vi "VisualizeTriggerTiming.vi"(1 "ExitExternalPrograms":refnum<notifier>, 2 "Pulse Settings":T1={"Pulse Length(ms)"=7.0, "DIO0Offset(ms)"=1.0, "DIO1 Pulse time (ms)"=2.0, "DIO2 Pulse time (ms) 2"=30.0, "DIO3 Pulse time (ms) 3"=0.0, "EnableDIO3"=FALSE, "EnableDIO2"=TRUE, "EnableDIO1"=TRUE}, 3 "Exposure Time (ms)":dbl=4.0, 4 "ReadoutTime":dbl=1.0, 5 "error in (no error)":errorcluster) -> (19 "error out":errorcluster)   [LabVIEW 2021]
doc: "This VI doest the same as DOconfigureCustomPattern but With a different Front panel. It is custom-made for the IAF Cytometer application"
uses:
  AD2_WFG_SDK_class/AD2TriggerSources.ctl
  AD2_SDK_class/AD2_SDK.lvclass
panel:
  in  "Tab Control":enum32{"Helper", "Ilustration"}(tab)
  out "Waveform Graph":dbl[][](graph)=[[0.0, 0.0, 0.0, 1.0, 1.0, 1.0, 1.0, 1.0, 1.0, 1.0, 0.0, 0.0, 0.0, 0.0, 0.0, 0.0, 0.0, 0.0, 0.0, 0.0, 0.0, 0.0, 0.0, 0.0, 0.0, 0.0, 0.0, 0.0, 0.0, 0.0, 0.0, 1.0, 1.0, 1.0, 1.0, 1.0, 1.0, 1.0, 0.0, 0.0, 0.0, 0.0, 0.0, 0.0], [0.0, 0.0, 1.1, 1.1, 1.1, 1.1, 1.1, 1.1, 1.1, 0.0, 0.0, 0.0, 0.0, 0.0, 0.0, 0.0, 0.0, 0.0, 0.0, 0.0, 0.0, 0.0, 0.0, 0.0, 0.0, 0.0, 0.0, 0.0, 0.0, 0.0, 0.0, 0.0, 0.0, 0.0, 0.0, 0.0, 0.0, 0.0, 0.0, 0.0, 0.0, 0.0, 0.0, 0.0], [0.0, 0.0, 0.0, 0.0, 0.0, 0.0, 0.0, 0.0, 0.0, 0.0, 0.0, 0.0, 0.0, 0.0, 0.0, 0.0, 0.0, 0.0, 0.0, 0.0, 0.0, 0.0, 0.0, 0.0, 0.0, 0.0, 0.0, 0.0, 0.0, 0.0, 1.2, 1.2, 1.2, 1.2, 1.2, 1.2, 1.2, 0.0, 0.0, 0.0, 0.0, 0.0, 0.0, 0.0], [0.0, 0.0, 0.0, 0.0, 0.0, 0.0, 0.0, 0.0, 0.0, 0.0, 0.0, 0.0, 0.0, 0.0, 0.0, 0.0, 0.0, 0.0, 0.0, 0.0, 0.0, 0.0, 0.0, 0.0, 0.0, 0.0, 0.0, 0.0, 0.0, 0.0, 0.0, 0.0, 0.0, 0.0, 0.0, 0.0, 0.0, 0.0, 0.0, 0.0, 0.0, 0.0, 0.0, 0.0], [0.0, 0.0, 0.0, 1.4, 1.4, 1.4, 1.4, 0.0, 0.0, 0.0, 0.0, 0.0, 0.0, 0.0, 0.0, 0.0, 0.0, 0.0, 0.0, 0.0, 0.0, 0.0, 0.0, 0.0, 0.0, 0.0, 0.0, 0.0, 0.0, 0.0, 0.0, 1.4, 1.4, 1.4, 1.4, 0.0, 0.0, 0.0, 0.0, 0.0, 0.0, 0.0, 0.0, 0.0], [0.0, 0.0, 0.0, 0.0, 0.0, 0.0, 0.0, 1.5, 0.0, 0.0, 0.0, 0.0, 0.0, 0.0, 0.0, 0.0, 0.0, 0.0, 0.0, 0.0, 0.0, 0.0, 0.0, 0.0, 0.0, 0.0, 0.0, 0.0, 0.0, 0.0, 0.0, 0.0, 0.0, 0.0, 0.0, 1.5, 0.0, 0.0, 0.0, 0.0, 0.0, 0.0, 0.0, 0.0]]
  out "appended array":bool[][](array[boolean])=[[FALSE, FALSE, FALSE, TRUE, TRUE, TRUE, TRUE, TRUE, TRUE, TRUE, FALSE, FALSE, FALSE, FALSE, FALSE, FALSE, FALSE, FALSE, FALSE, FALSE, FALSE, FALSE, FALSE, FALSE, FALSE, FALSE, FALSE, FALSE, FALSE, FALSE, FALSE, TRUE, TRUE, TRUE, TRUE, TRUE, TRUE, TRUE, FALSE, FALSE, FALSE, FALSE, FALSE, FALSE], [FALSE, FALSE, TRUE, TRUE, TRUE, TRUE, TRUE, TRUE, TRUE, FALSE, FALSE, FALSE, FALSE, FALSE, FALSE, FALSE, FALSE, FALSE, FALSE, FALSE, FALSE, FALSE, FALSE, FALSE, FALSE, FALSE, FALSE, FALSE, FALSE, FALSE, FALSE, FALSE, FALSE, FALSE, FALSE, FALSE, FALSE, FALSE, FALSE, FALSE, FALSE, FALSE, FALSE, FALSE], [FALSE, FALSE, FALSE, FALSE, FALSE, FALSE, FALSE, FALSE, FALSE, FALSE, FALSE, FALSE, FALSE, FALSE, FALSE, FALSE, FALSE, FALSE, FALSE, FALSE, FALSE, FALSE, FALSE, FALSE, FALSE, FALSE, FALSE, FALSE, FALSE, FALSE, TRUE, TRUE, TRUE, TRUE, TRUE, TRUE, TRUE, FALSE, FALSE, FALSE, FALSE, FALSE, FALSE, FALSE], [FALSE, FALSE, FALSE, FALSE, FALSE, FALSE, FALSE, FALSE, FALSE, FALSE, FALSE, FALSE, FALSE, FALSE, FALSE, FALSE, FALSE, FALSE, FALSE, FALSE, FALSE, FALSE, FALSE, FALSE, FALSE, FALSE, FALSE, FALSE, FALSE, FALSE, FALSE, FALSE, FALSE, FALSE, FALSE, FALSE, FALSE, FALSE, FALSE, FALSE, FALSE, FALSE, FALSE, FALSE], [FALSE, FALSE, FALSE, TRUE, TRUE, TRUE, TRUE, FALSE, FALSE, FALSE, FALSE, FALSE, FALSE, FALSE, FALSE, FALSE, FALSE, FALSE, FALSE, FALSE, FALSE, FALSE, FALSE, FALSE, FALSE, FALSE, FALSE, FALSE, FALSE, FALSE, FALSE, TRUE, TRUE, TRUE, TRUE, FALSE, FALSE, FALSE, FALSE, FALSE, FALSE, FALSE, FALSE, FALSE], [FALSE, FALSE, FALSE, FALSE, FALSE, FALSE, FALSE, TRUE, FALSE, FALSE, FALSE, FALSE, FALSE, FALSE, FALSE, FALSE, FALSE, FALSE, FALSE, FALSE, FALSE, FALSE, FALSE, FALSE, FALSE, FALSE, FALSE, FALSE, FALSE, FALSE, FALSE, FALSE, FALSE, FALSE, FALSE, TRUE, FALSE, FALSE, FALSE, FALSE, FALSE, FALSE, FALSE, FALSE]]
  in  "Exit Pulse Helper":bool
  # "DIO0 Pulses at the same time as DIO1,2 and 3 +-offset\nSet Pulse Length > exposure time+readout time"
  # "DIO0 (camera)"
  # "DIO1 (COOL-LED CH1)"
  # "DIO2 (COOL-LED CH2)"
  # "DIO3 (COOL-LED CH3)"
  # "Each Element is 1ms"
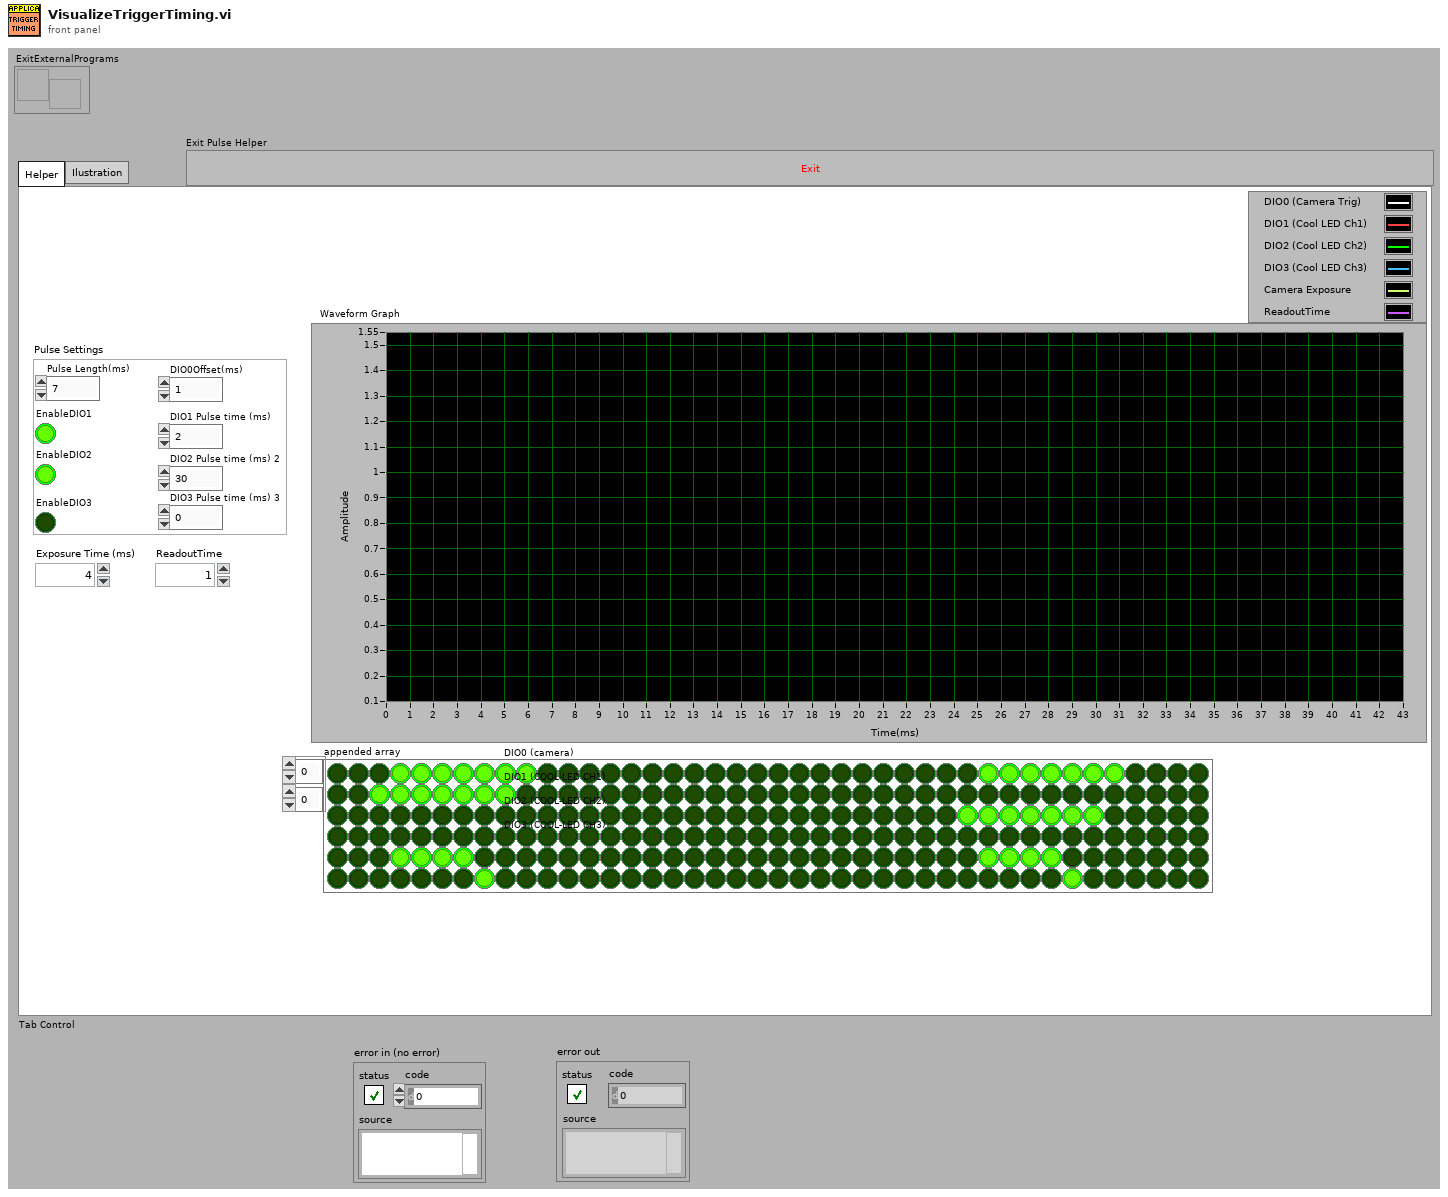
[diagram p1: front panel]
types:
  T1 = cluster{"Pulse Length(ms)":dbl, "DIO0Offset(ms)":dbl, "DIO1 Pulse time (ms)":dbl, "DIO2 Pulse time (ms) 2":dbl, "DIO3 Pulse time (ms) 3":dbl, "EnableDIO3":bool, "EnableDIO2":bool, "EnableDIO1":bool}
  T2 = typedef "AD2_SDK.lvclass/AD2TriggerSources.ctl" = enum8{"trigrsrcNone", "trigsrcPC", "trigsrcDetectorAnalogIn", "trigsrcDetectorDigitalIn", "trigsrcAnalogIn", "trigsrcDigitalIn", "trigsrcDigitalOut", "trigsrcAnalogOut1", "trigsrcAnalogOut2", "trigsrcAnalogOut3", "trigsrcAnalogOut4", "trigsrcExternal1", "trigsrcExternal2", "trigsrcExternal3", "trigsrcExternal4", ""}
  T3 = cluster{"Data":bool[], "Freq":dbl, "#Bits":u32, "Enable":bool}[]
  T4 = cluster{"secRun(0=Cont)":dbl, "secWait":dbl, "cRepeat(0=inf)":i32, "Repeat Trigger":bool, "TrigrSrc":T2}
  T5 = cluster{"Data":bool[], "Freq":dbl, "#Bits":u32, "Enable":bool}
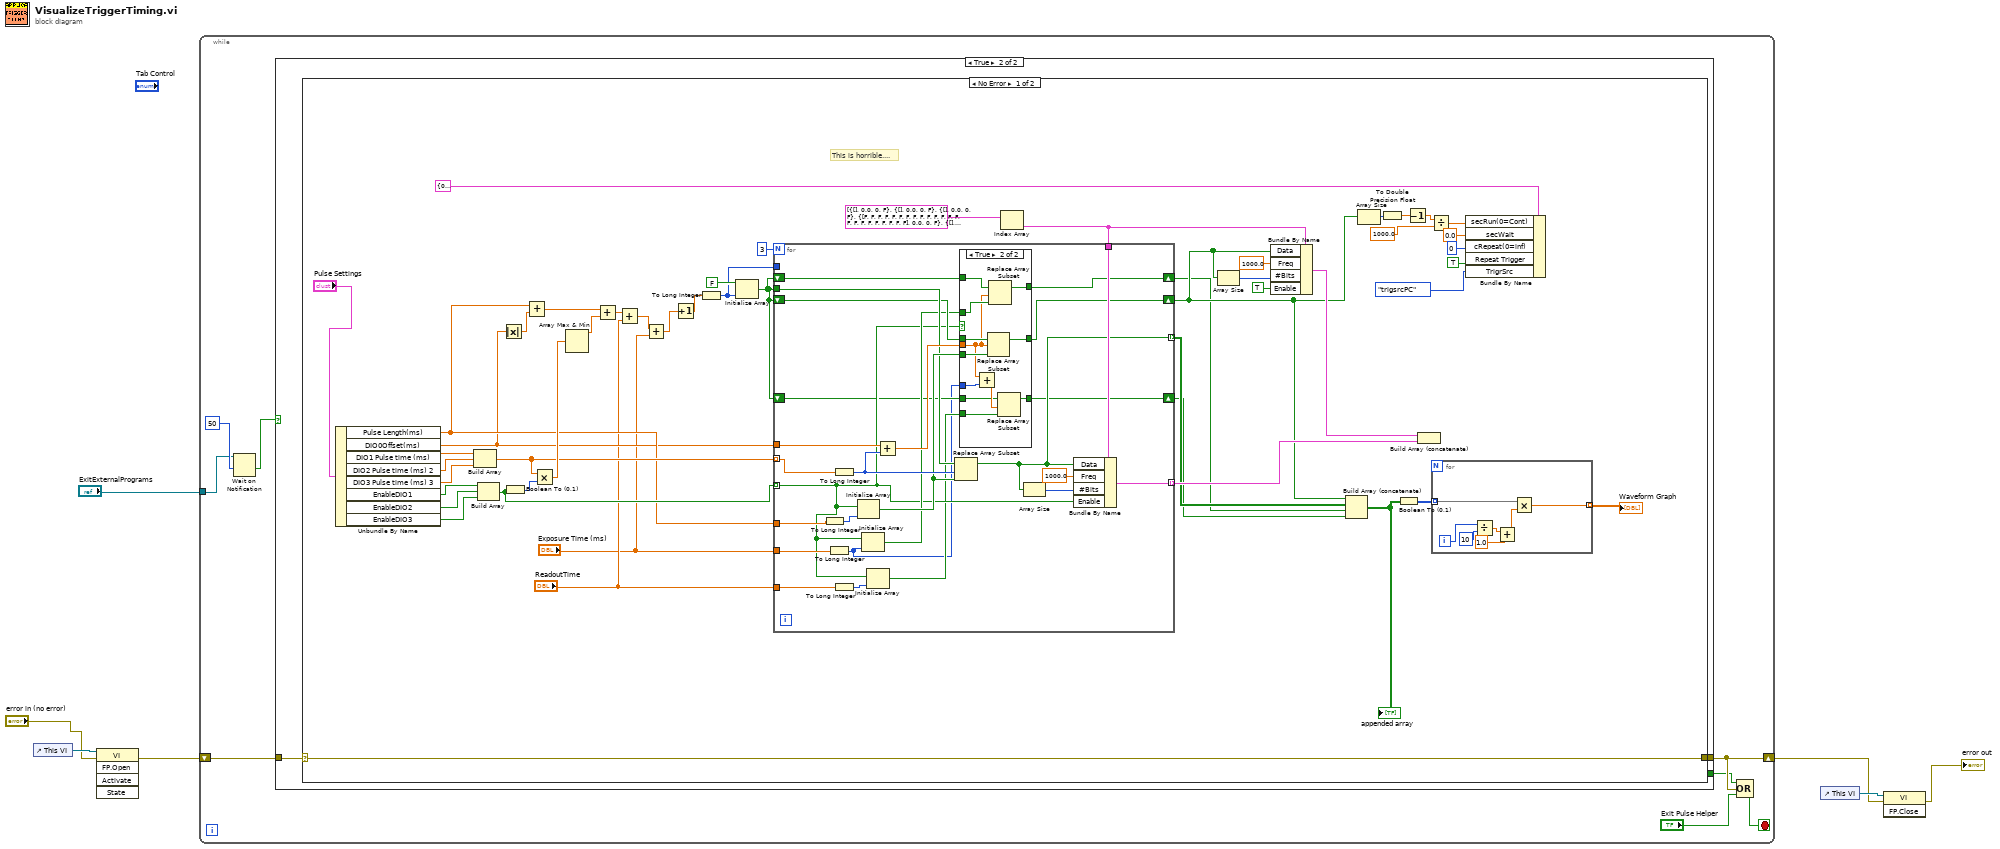
[diagram p0: block diagram]
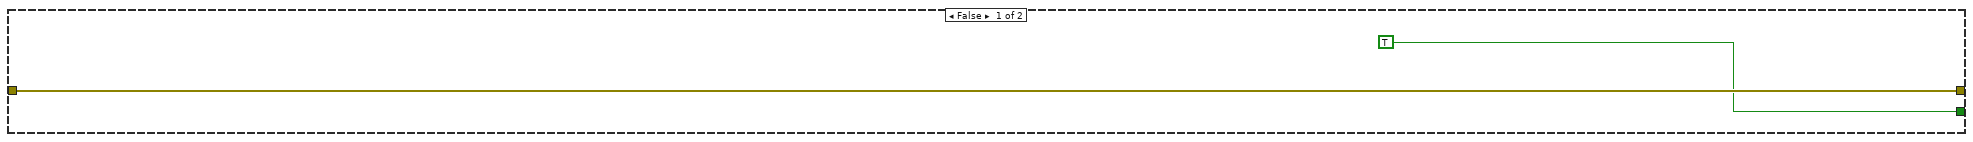
[diagram p2: hidden frame]
diagram:
  n1 = control-ref of="This VI"() -> (w4:refnum<vi>)
  n2 = invoke class="VI" method="FP.Open"(reference=w4, error in="error in (no error)") -> (error out=w2:errorcluster)  [unwired: 3 in, 4 out]
  n3 = while {
    shift-right: [w9] -> w6
    shift-left: w2 -> [w15]
    tunnel: "ExitExternalPrograms" -> [w13]
    stop <- w10 stop-if-true
    n4 = Wait on Notification(notifier=w13, timeout in ms (-1)=u32 50 ("millisecond multiple")) -> (timed out?=w12:bool)  [unwired: 2 in, 3 out]
    n5 = case shown="True" w12 {
      tunnel: w15 -> [w17 w19]
      tunnel: [w17 w18] -> w9
      tunnel: [TRUE _] -> w8
      frame False {
      }
      frame True {
        n6 = case shown="No Error" w19 {
          selector: w19 -> [w34 w119]
          tunnel: [w34 w119] -> w18
          frame No Error {
            # "This is horrible...."
            n7 = Unbundle By Name("Pulse Settings") -> ("Pulse Length(ms)"=w53:dbl, "DIO0Offset(ms)"=w51:dbl, "DIO1 Pulse time (ms)"=w54:dbl, "DIO2 Pulse time (ms) 2"=w63:dbl, "DIO3 Pulse time (ms) 3"=w62:dbl, "EnableDIO1"=w66:bool, "EnableDIO2"=w65:bool, "EnableDIO3"=w64:bool)
            n8 = Build Array(w54, w63, w62) -> (w57:dbl[])
            n9 = Build Array(w66, w65, w64) -> (w56:bool[])
            n10 = Absolute Value(x=w51) -> (abs(x)=w50:dbl)
            n11 = Boolean To (0,1)(Boolean=w56) -> (0, 1=w61:i16[])
            n12 = Add(x=w53, y=w50) -> (x+y=w52:dbl)
            n13 = Multiply(x=w57, y=w61) -> (x*y=w60:dbl[])
            n14 = Array Max & Min(array=w60) -> (max value=w59:dbl)  [unwired: 3 out]
            n15 = Add(x=w52, y=w59) -> (x+y=w23:dbl)
            n16 = Add(x=w23, y="ReadoutTime") -> (x+y=w22:dbl)
            n17 = Add(x=w22, y="Exposure Time (ms)") -> (x+y=w21:dbl)
            n18 = Increment(x=w21) -> (x+1=w36:dbl)
            n19 = To Long Integer(number=w36) -> (32bit integer=w46:i32)
            n20 = Initialize Array(FALSE, w46) -> (w26:bool[])
            n21 = Index Array(array=T3 [{"Data"=[], "Freq"=0.0, "#Bits"=0, "Enable"=FALSE}, {"Data"=[], "Freq"=0.0, "#Bits"=0, "Enable"=FALSE}, {"Data"=[], "Freq"=0.0, "#Bits"=0, "Enable"=FALSE}, {"Data"=[FALSE, FALSE, FALSE, FALSE, FALSE, FALSE, FALSE, FALSE, FALSE, FALSE, FALSE, FALSE, FALSE, FALSE, FALSE, FALSE, FALSE, FALSE, FALSE, FALSE, FALSE, FALSE, FALSE], "Freq"=0.0, "#Bits"=0, "Enable"=FALSE}, {"Data"=[], "Freq"=0.0, "#Bits"=0, "Enable"=FALSE}, {"Data"=[], "Freq"=0.0, "#Bits"=0, "Enable"=FALSE}, {"Data"=[], "Freq"=0.0, "#Bits"=0, "Enable"=FALSE}, {"Data"=[], "Freq"=0.0, "#Bits"=0, "Enable"=FALSE}, {"Data"=[], "Freq"=0.0, "#Bits"=0, "Enable"=FALSE}, {"Data"=[], "Freq"=0.0, "#Bits"=0, "Enable"=FALSE}, {"Data"=[], "Freq"=0.0, "#Bits"=0, "Enable"=FALSE}, {"Data"=[], "Freq"=0.0, "#Bits"=0, "Enable"=FALSE}, {"Data"=[], "Freq"=0.0, "#Bits"=0, "Enable"=FALSE}, {"Data"=[], "Freq"=0.0, "#Bits"=0, "Enable"=FALSE}, {"Data"=[], "Freq"=0.0, "#Bits"=0, "Enable"=FALSE}, {"Data"=[FALSE, FALSE, FALSE, FALSE, FALSE, FALSE, FALSE, FALSE, FALSE, FALSE, FALSE, FALSE, FALSE, FALSE, FALSE, FALSE, FALSE, FALSE, FALSE, FALSE, FALSE, FALSE, FALSE], "Freq"=0.0, "#Bits"=0, "Enable"=FALSE}, {"Data"=[FALSE, FALSE, FALSE, FALSE, FALSE, FALSE, FALSE, FALSE, FALSE, FALSE, FALSE, FALSE, FALSE, FALSE, FALSE, FALSE, FALSE, FALSE, FALSE, FALSE, FALSE, FALSE, FALSE], "Freq"=0.0, "#Bits"=0, "Enable"=FALSE}] ("CustomData")) -> (element=w45:T5)  [unwired: 1 in]
            n22 = for {
              N: 3 -> [_]
              tunnel: w45 -> [w95]
              tunnel: w57 -> [w89] mode=indexing
              tunnel: w56 -> [w84] mode=indexing
              tunnel: w53 -> [w103]
              tunnel: w26 -> [w97]
              shift-right: [w94] -> w33
              shift-left: w26 -> [w96]
              tunnel: w51 -> [w100]
              tunnel: w46 -> [_]
              tunnel: [w92] -> w40 mode=indexing
              tunnel: [w90] -> w32 mode=indexing
              tunnel: "Exposure Time (ms)" -> [w88]
              shift-right: [w86] -> w27
              shift-left: w26 -> [w85]
              tunnel: "ReadoutTime" -> [w83]
              shift-right: [w80] -> w25
              shift-left: w26 -> [w81]
              n23 = To Long Integer(number=w103) -> (32bit integer=w102:i32)
              n24 = To Long Integer(number=w88) -> (32bit integer=w79:i32)
              n25 = To Long Integer(number=w89) -> (32bit integer=w101:i32)
              n26 = To Long Integer(number=w83) -> (32bit integer=w78:i32)
              n27 = Initialize Array(w84, w102) -> (w98:bool[])
              n28 = Initialize Array(w84, w79) -> (w87:bool[])
              n29 = Initialize Array(w84, w78) -> (w82:bool[])
              n30 = Add(x=w100, y=w101) -> (x+y=w99:dbl)
              n31 = Replace Array Subset(array=w97, new element=w98, index=w101) -> (w90:bool[])
              n32 = case shown="True" w84 {
                tunnel: w99 -> [_ w112]
                tunnel: w98 -> [_ w118]
                tunnel: w96 -> [w106 w116]
                tunnel: [w106 w117] -> w94
                tunnel: w87 -> [_ w115]
                tunnel: [w105 w114] -> w86
                tunnel: w85 -> [w105 w113]
                tunnel: w79 -> [_ w111]
                tunnel: w82 -> [_ w109]
                tunnel: w81 -> [w104 w108]
                tunnel: [w104 w107] -> w80
                frame False {
                }
                frame True {
                  n33 = Add(x=w112, y=w111) -> (x+y=w110:dbl)
                  n34 = Replace Array Subset(array=w116, new element=w118, index=w112) -> (w117:bool[])
                  n35 = Replace Array Subset(array=w113, new element=w115, index=w112) -> (w114:bool[])
                  n36 = Replace Array Subset(array=w108, new element=w109, index=w110) -> (w107:bool[])
                }
              }
              n37 = Array Size(array=w90) -> (size(s)=w91:i32)
              n38 = Bundle By Name(cluster=w95, "Data"=w90, "Freq"=1000.0, "#Bits"=w91, "Enable"=w84) -> (w92:T5)
            }
            n39 = Array Size(array=w33) -> (size(s)=w43:i32)
            n40 = Bundle By Name(cluster=w45, "Data"=w33, "Freq"=1000.0, "#Bits"=w43, "Enable"=TRUE) -> (w41:T5)
            n41 = Build Array (concatenate)(w33, w32, w27, w25) -> (w31:bool[][])
            "appended array" <- w31
            n42 = Array Size(array=w33) -> (size(s)=w47:i32)
            n43 = To Double Precision Float(number=w47) -> (double precision float=w38:dbl)
            n44 = Boolean To (0,1)(Boolean=w31) -> (0, 1=w30:i16[][])
            n45 = Decrement(x=w38) -> (x-1=w37:dbl)
            n46 = Build Array (concatenate)(w41, w40) -> ()  [unwired: 1 out]
            n47 = Divide(x=w37, y=1000.0) -> (x/y=w48:dbl)
            n48 = for {
              tunnel: w30 -> [w76] mode=indexing
              tunnel: [w75] -> w29 mode=indexing
              i -> [w74]
              n49 = Divide(x=w74, y=10) -> (x/y=w73:dbl)
              n50 = Add(x=w73, y=1.0) -> (x+y=w72:dbl)
              n51 = Multiply(x=w76, y=w72) -> (x*y=w75:dbl[])
            }
            "Waveform Graph" <- w29
            n52 = Bundle By Name(cluster=T4 {"secRun(0=Cont)"=0.0, "secWait"=0.0, "cRepeat(0=inf)"=0, "Repeat Trigger"=FALSE, "TrigrSrc"=enum."trigrsrcNone"} ("DO Trigger"), "secRun(0=Cont)"=w48, "secWait"=0.0, "cRepeat(0=inf)"=0, "Repeat Trigger"=TRUE, "TrigrSrc"=AD2TriggerSources."trigsrcPC") -> ()  [unwired: 1 out]
          }
          frame Error {
          }
        }
      }
    }
    n53 = Compound Arithmetic op=OR(w8, w9, "Exit Pulse Helper") -> (w10:bool)
  }
  n54 = control-ref of="This VI"() -> (w7:refnum<vi>)
  n55 = invoke class="VI" method="FP.Close"(reference=w7, error in=w6) -> (error out=→"error out":errorcluster)  [unwired: 1 in, 2 out]
